vi "Check if Confirmed.vi"(8 "error in":errorcluster, 9 "Request Tick":u32, 10 "Node ID":u8, 11 "Node Guard in":refnum<class "Node Guard.lvclass">) -> (0 "error out":errorcluster, 3 "Node Guard out":refnum<class "Node Guard.lvclass">)   [LabVIEW 2020, in "CANopen.lvlib" / "Network Management.lvlib" / "Node Guard.lvlib" / "Node Guard.lvclass"]
uses:
  Node Guard.lvclass
  C:/Program Files/National Instruments/LabVIEW 2026/vi.lib/ActorFramework/Actor/Actor.lvclass
  Node Guard Messages/Check if Confirmed Msg/Check if Confirmed Msg.lvclass
  C:/Program Files/National Instruments/LabVIEW 2026/vi.lib/ActorFramework/Message/Message.lvclass
  <vilib>/ActorFramework/Actor/Actor.lvclass/Actor.ctl
  <vilib>/ActorFramework/Message Enqueuer/Message Enqueuer.lvclass/Message Enqueuer.ctl
  Node Guard.lvclass/Node Guard.ctl
  Node Guard Messages/Check if Confirmed Msg/Check if Confirmed Msg.lvclass/Check if Confirmed Msg.ctl
  <vilib>/ActorFramework/Message Enqueuer/Message Enqueuer.lvclass
  <vilib>/ActorFramework/Actor Framework.lvlib
  <vilib>/ActorFramework/Actor/Actor.lvclass
  <vilib>/ActorFramework/Time-Delayed Send Message/Time-Delay Override Options.ctl
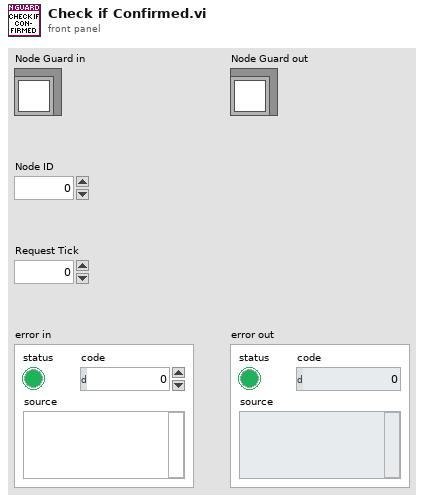
[diagram p1: front panel]
types:
  T1 = cluster{"State":u8, "Timings":cluster{"Guard time (ms)":u32, "Lifetime Factor":dbl}, "Toogle Bit":bool, "Delivery Notifier":refnum<notifier>, "Last Received Tick":u32}
  T2 = map{u8, cluster{"State":u8, "Timings":cluster{"Guard time (ms)":u16, "Lifetime Factor":u8}, "Toogle Bit":bool, "Delivery Notifier":refnum<notifier>, "Last Received Tick":u32}}
  T3 = cluster{"State":u8, "Timings":cluster{"Guard time (ms)":u16, "Lifetime Factor":u8}, "Toogle Bit":bool, "Delivery Notifier":refnum<notifier>, "Last Received Tick":u32}
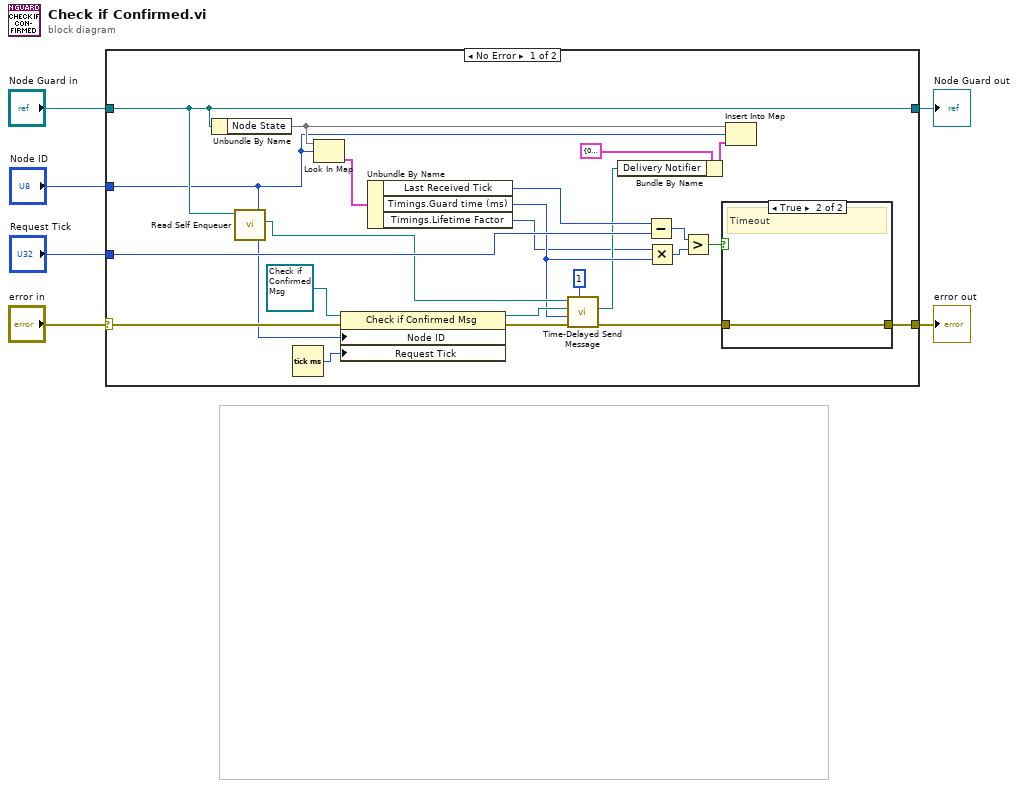
[diagram p0: block diagram]
diagram:
  n1 = case shown="No Error" "error in" {
    selector: "error in" -> [w21 w33]
    tunnel: [w15 w33] -> w3
    tunnel: [w18 w32] -> w5
    tunnel: "Node Guard in" -> [w18 w32]
    tunnel: "Node ID" -> [w12 _]
    tunnel: "Request Tick" -> [w27 _]
    frame No Error {
      n2 = Unbundle By Name(w18) -> ("Node State"=w13:T2)
      n3 = call <vilib>:"Read Self Enqueuer.vi"("Actor"=w18) -> ("Self Enqueuer"=w19:refnum<class "Message Enqueuer.lvclass">)  [unwired: 10 in]
      n4 = Tick Count (ms)() -> (millisecond timer value=w20:u32)
      n5 = Look In Map(map=w13, key=w12) -> (value=w29:T3)  [unwired: 1 in, 1 out]
      n6 = property class="Check if Confirmed Msg"(reference=refnum<class "Check if Confirmed Msg.lvclass"> refnum ("CANopen.lvlib:Node Guard.lvlib:Check if Confirmed Msg.lvclass"), error in=w21, "Node ID"=w12, "Request Tick"=w20) -> (reference out=w23:refnum<class "Check if Confirmed Msg.lvclass">, error out=w22:errorcluster)
      n7 = Unbundle By Name(w29) -> ("Last Received Tick"=w28:u32, "Timings.Guard time (ms)"=w17:u16, "Timings.Lifetime Factor"=w7:u8)
      n8 = call <vilib>:"Time-Delayed Send Message.vi"("# Copies (0 = infinite repeat)"=u32 1, "error in (no error)"=w22, "Milliseconds To Wait"=w17, "Message"=w23, "Message Enqueuer"=w19) -> ("error out"=w16:errorcluster, "Delivery Notifier"=w9:refnum<notifier>)  [unwired: 5 in]
      n9 = Bundle By Name(cluster=T1 {"State"=0, "Timings"={"Guard time (ms)"=0, "Lifetime Factor"=0.0}, "Toogle Bit"=FALSE, "Delivery Notifier"=refnum, "Last Received Tick"=0} ("value"), "Delivery Notifier"=w9) -> (w10:T1)
      n10 = Subtract(x=w28, y=w27) -> (x-y=w26:u32)
      n11 = Multiply(x=w7, y=w17) -> (x*y=w8:u16)
      n12 = Greater?(x=w26, y=w8) -> (0:w14:bool)
      n13 = case shown="True" w14 {
        tunnel: [w30 w31] -> w15
        tunnel: w16 -> [w30 w31]
        frame False {
        }
        frame True {
          # "Timeout"
        }
      }
      n14 = Insert Into Map(map in=w13, key=w12, value=w10) -> ()  [unwired: 3 out]
    }
    frame Error {
    }
  }
  "Node Guard out" <- w5
  "error out" <- w3
